vi "NewVision.vi"   [LabVIEW 2018]
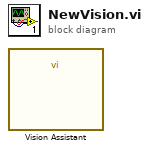
[diagram p0: block diagram]
diagram:
  n1 = call "Vision Assistant"() -> ()  [unwired: 26 in, 2 out]
